vi "Écrire Stocks.vi"(10 "Stocks":refnum<class "Stock.lvclass">[](array[class]), 11 "Portfolio en entrée":refnum<class "Portfolio.lvclass">) -> (3 "Portfolio en sortie":refnum<class "Portfolio.lvclass">)   [LabVIEW 2012, in "Portfolio.lvclass"]
uses:
  Portfolio.lvclass
  Stock/Stock.lvclass
  Portfolio.lvclass/Portfolio.ctl
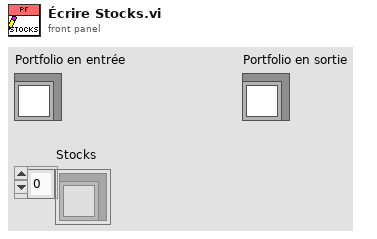
[diagram p1: front panel]
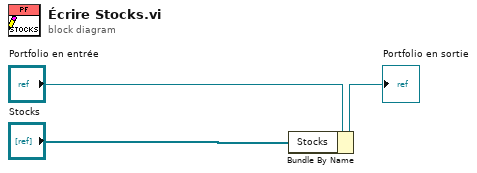
[diagram p0: block diagram]
diagram:
  n1 = Bundle By Name(cluster="Portfolio en entrée", "Stocks"="Stocks") -> (→"Portfolio en sortie":refnum<class "Portfolio.lvclass">)
